vi "Read Is Server.vi"(8 "error in (no error)":errorcluster, 11 "WebSocket Server in":refnum<class "WebSocket Server.lvclass">) -> (0 "error out":errorcluster, 2 "Is Server?":bool, 3 "WebSocket Server out":refnum<class "WebSocket Server.lvclass">)   [LabVIEW 2021, in "WebSockets.lvlib" / "WebSocket Server.lvclass"]
doc: "WebSockets 2.0.1.40\nSam Sharp - MediaMongrels Ltd\nCopyright (c) 2019, MediaMongrels Ltd"
uses:
  WebSocket Server.lvclass
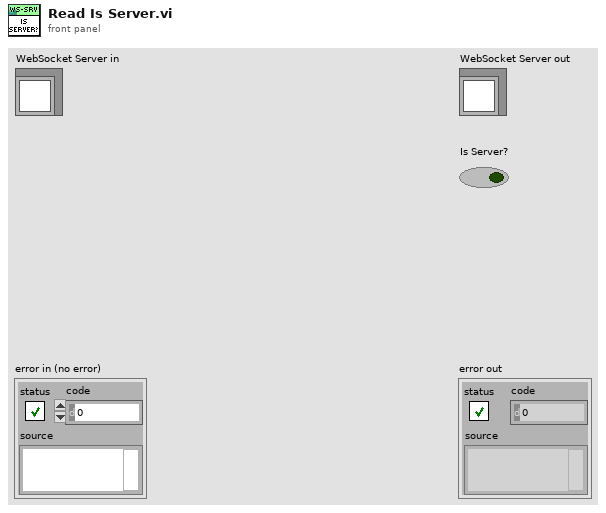
[diagram p1: front panel]
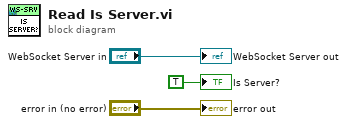
[diagram p0: block diagram]
diagram:
  "error out" <- "error in (no error)"
  "WebSocket Server out" <- "WebSocket Server in"
  "Is Server?" <- TRUE ("Is Server?")
